vi "TA_Generate_DelayTime_LinearExponential.vi"(8 "Exponential\nNumber of Steps":dbl[](array[numeric])=[100.0, 100.0, 100.0, 100.0], 9 "Exponential \nTime Range (ps)":dbl[](array[numeric])=[1.0, 10.0, 100.0, 1000.0, 10000.0], 10 "Linear\nStep (ps)":dbl[](array[numeric])=[0.5, 0.05], 11 "Linear \nTime Range (ps)":dbl[](array[numeric])=[-10.0, -1.0, 1.0]) -> (2 "Number (Delay Time)":i32, 3 "Generated Delay Time (ps)":dbl[](array[numeric]))   [LabVIEW 2025]
uses:
  <vilib>/Analysis/NI_AALBase.lvlib
  <vilib>/Analysis/1siggen.llb/Ramp Pattern by Delta.vi
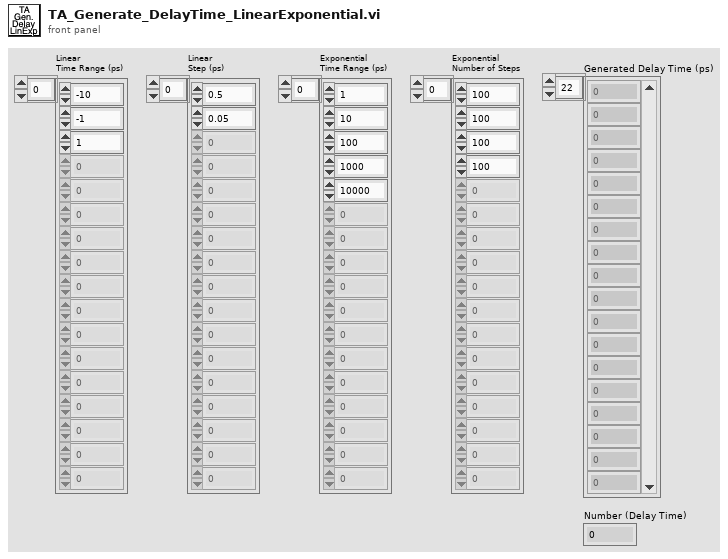
[diagram p1: front panel]
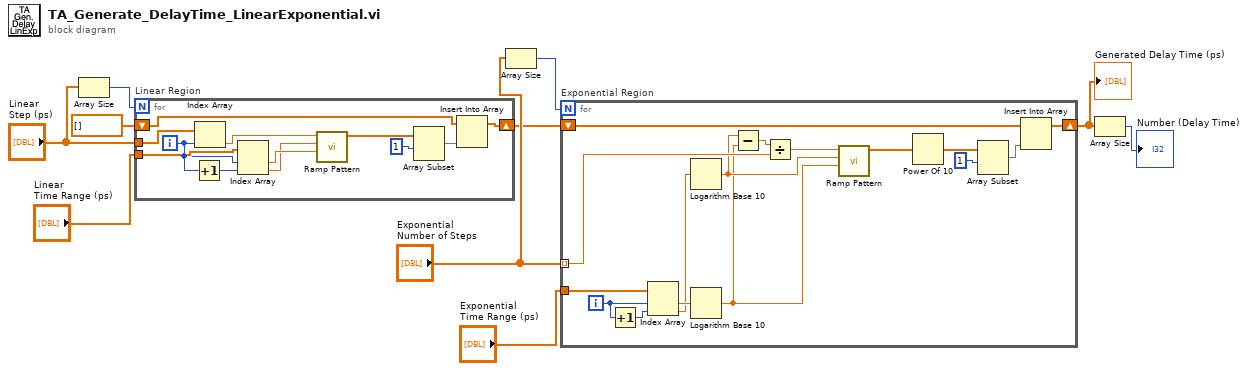
[diagram p0: block diagram]
diagram:
  n1 = Array Size(array="Linear\nStep (ps)") -> (size(s)=w9:i32)
  n2 = for "Linear Region" {
    N: w9 -> [_]
    tunnel: "Linear \nTime Range (ps)" -> [w22]
    tunnel: "Linear\nStep (ps)" -> [w18]
    shift-right: [w14] -> w2
    shift-left: dbl[] [] ("Array") -> [w15]
    i -> [w16]
    n3 = Increment(x=w16) -> (x+1=w21:i32)
    n4 = Index Array(array=w18, index=w16) -> (element=w17:dbl)
    n5 = Index Array(array=w22, index #1=w16, index #2=w21) -> (element #1=w20:dbl, element #2=w19:dbl)
    n6 = call-poly <vilib>:"Ramp Pattern.vi"("start"=w20, "end"=w19, "delta"=w17) -> ("Ramp Pattern"=w13:dbl[])  [unwired: 6 in, 2 out]
    n7 = Array Subset(array=w13, index=1) -> (w11:dbl[])  [unwired: 1 in]
    n8 = Insert Into Array(array=w15, new element=w11) -> (w14:dbl[])  [unwired: 1 in]
  }
  n9 = Array Size(array="Exponential\nNumber of Steps") -> (size(s)=w4:i32)
  n10 = for "Exponential Region" {
    N: w4 -> [_]
    tunnel: "Exponential \nTime Range (ps)" -> [w38]
    tunnel: "Exponential\nNumber of Steps" -> [w32] mode=indexing
    shift-right: [w34] -> w1
    shift-left: w2 -> [w35]
    i -> [w37]
    n11 = Increment(x=w37) -> (x+1=w36:i32)
    n12 = Index Array(array=w38, index #1=w37, index #2=w36) -> (element #1=w30:dbl, element #2=w29:dbl)
    n13 = Logarithm Base 10(1:w29) -> (0:w28:dbl)
    n14 = Logarithm Base 10(1:w30) -> (0:w27:dbl)
    n15 = Subtract(x=w28, y=w27) -> (x-y=w33:dbl)
    n16 = Divide(x=w33, y=w32) -> (x/y=w31:dbl)
    n17 = call-poly <vilib>:"Ramp Pattern.vi"("start"=w27, "end"=w28, "delta"=w31) -> ("Ramp Pattern"=w26:dbl[])  [unwired: 6 in, 2 out]
    n18 = Power Of 10(x=w26) -> (10^x=w25:dbl[])
    n19 = Array Subset(array=w25, index=1) -> (w23:dbl[])  [unwired: 1 in]
    n20 = Insert Into Array(array=w35, new element=w23) -> (w34:dbl[])  [unwired: 1 in]
  }
  "Generated Delay Time (ps)" <- w1
  n21 = Array Size(array=w1) -> (size(s)=→"Number (Delay Time)":i32)
